vi "Read Hand Position Velocity.vi"   [LabVIEW 2011, in "LVH-Leap.lvlib"]
uses:
  LVH-Leap.lvlib
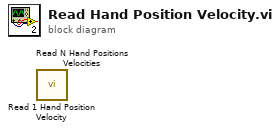
[diagram p0: block diagram]
diagram:
  n1 = call "Read 1 Hand Position Velocity.vi"() -> ()  [unwired: 8 in, 4 out]
  n2 = call "Read N Hand Positions Velocities.vi"() -> ()  [unwired: 8 in, 4 out]
